vi "INI Read write DBL 1D storage.vi"(6 "Values to write":dbl[][](array[numeric]), 7 "Read/Write mode":T2, 8 "error in":errorcluster, 9 "Defaults":dbl[](array[numeric]), 10 "keys":string[](array[string]), 11 "Config file section":T1=enum."Exp (ms) per RO") -> (0 "error out":errorcluster, 2 "Values":dbl[][](array[numeric]))   [LabVIEW 2013]
doc: "This module is used to store and retrieve information from the .ini file. On first call, it reads from the file on disk and stores the information in memory."
uses:
  Read write mode.ctl
  Configuration INI file IO/Config file sections enum.ctl
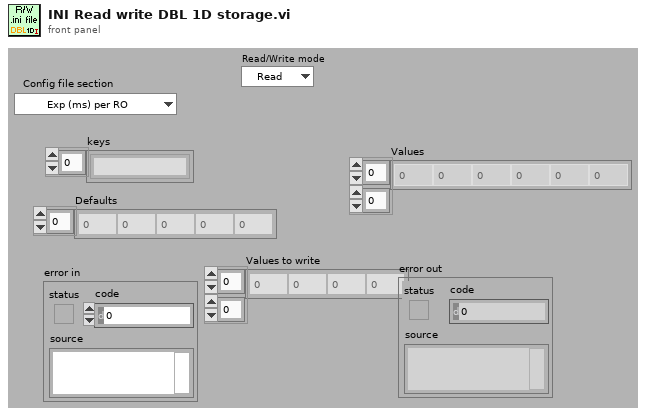
[diagram p1: front panel]
types:
  T1 = typedef "Config file sections enum.ctl" = enum16{"General config", "SLM", "Sequence setpoints", "Exp (ms) per RO", "2 Color"}
  T2 = typedef "Read write mode.ctl" = enum16{"Read", "Write"}
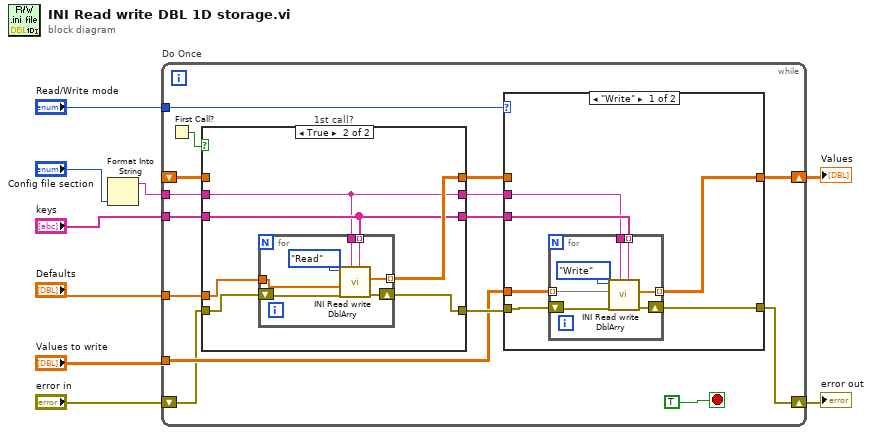
[diagram p0: block diagram]
diagram:
  n1 = Format Into String("Config file section") -> (resulting string=w2:string)  [unwired: 3 in, 1 out]
  n2 = while "Do Once" {
    tunnel: w2 -> [w22]
    tunnel: "Read/Write mode" -> [w21]
    tunnel: "Values to write" -> [w14]
    tunnel: "keys" -> [w16]
    shift-right: [w13] -> w8
    shift-left: _ -> [w15]
    tunnel: "Defaults" -> [w10]
    shift-right: [w11] -> w4
    shift-left: "error in" -> [w12]
    stop <- TRUE stop-if-true
    n3 = First Call?() -> (First Call?: T/F=w23:bool)
    n4 = case "1st call?" shown="True" w23 {
      tunnel: w22 -> [w43 w45]
      tunnel: w16 -> [w42 w48]
      tunnel: [w41 w49] -> w17
      tunnel: [w40 w44] -> w20
      tunnel: [w43 w45] -> w19
      tunnel: [w42 w48] -> w18
      tunnel: w15 -> [w41 _]
      tunnel: w12 -> [w40 w47]
      tunnel: w10 -> [_ w46]
      frame False {
      }
      frame True {
        n5 = for {
          tunnel: [w55] -> w49 mode=indexing
          shift-right: [w54] -> w44
          shift-left: w47 -> [w56]
          tunnel: w45 -> [w52]
          tunnel: w48 -> [w51] mode=indexing
          tunnel: w46 -> [w50]
          n6 = call "INI Read write DblArry.vi"("key"=w51, "section"=w52, "error in"=w56, "default"=w50, "Read|Write"=Read_write_mode."Read") -> ("error out"=w54:errorcluster, "dbl array out"=w55:dbl[])  [unwired: 5 in]
        }
      }
    }
    n7 = case "1st call?" shown="\"Write\"" w21 {
      tunnel: w20 -> [w30 w38]
      tunnel: w19 -> [w26 _]
      tunnel: w18 -> [w29 _]
      tunnel: [w28 w39] -> w13
      tunnel: [w25 w38] -> w11
      tunnel: w17 -> [_ w39]
      tunnel: w14 -> [w27 _]
      frame "Write" {
        n8 = for {
          shift-right: [w36] -> w25
          shift-left: w30 -> [w37]
          tunnel: w29 -> [w34] mode=indexing
          tunnel: w26 -> [w33]
          tunnel: w27 -> [w31] mode=indexing
          tunnel: [w32] -> w28 mode=indexing
          n9 = call "INI Read write DblArry.vi"("key"=w34, "section"=w33, "error in"=w37, "dbl array in"=w31, "Read|Write"=Read_write_mode."Write") -> ("error out"=w36:errorcluster, "dbl array out"=w32:dbl[])  [unwired: 5 in]
        }
      }
      frame "Read" {
      }
    }
  }
  "Values" <- w8
  "error out" <- w4
